vi "mod_Continuous BB-PSK generation.vi"(0 "bit stream type":T4(tab), 1 "Symbol Rate, Hz":dbl=1.0 format="%.2f", 2 "Custom-PSK Parameters":T3 {"PSK type" items=["normal", "shifted", "offset"]; "symbol map" format="%.3f"}, 5 "PN Sequence Order":i32=9, 9 "user base bit pattern":i8[](array[numeric]), 11 "error in (no error)":errorcluster, 12 "filter parameters":T1={"Alpha"=0.5, "Filter Length"=6, "TX Filter"=enum."Root Raised Cos"} {"Alpha" format="%.2f"}, 13 "Path":path) -> (4 "output complex waveform":T2 {"Y" format="%.3f"; "dt" format="%^.2e"; "t0" format="%.4f"}, 6 "samples per symbol":i32, 15 "error out":errorcluster)   [LabVIEW 2020, in "niDMT.lvlib"]
uses:
  <vilib>/addons/Modulation/niDMT.lvlib
  <vilib>/addons/Modulation/Digital/Support/Controls/PSK System Parameters.ctl
  <vilib>/addons/Modulation/Analog/controls/Complex Data Waveform.ctl
  <vilib>/addons/Modulation/Digital/General/MT Generate Bits (Galois, PN Order).vi
  <vilib>/addons/Modulation/Digital/Support/Common/Validators/mod_Generate Bits Validate.vi
  <vilib>/addons/Modulation/Analog/support/mod_Set Error Source.vi
  <vilib>/addons/Modulation/Digital/General/subVIs/mod_Generate Bits PN Sequence.vi
  <vilib>/addons/Modulation/Digital/General/MT Generate Bits (User Defined).vi
  <vilib>/Utility/file.llb/Read From Spreadsheet File (DBL).vi
  <vilib>/addons/Modulation/Digital/Support/Common/Validators/mod_Generate Filter Coefficients Validate.vi
  <vilib>/addons/Modulation/Digital/General/subVIs/mod_Generate Filter Coefficients.vi
  <vilib>/addons/Modulation/niAMT.lvlib
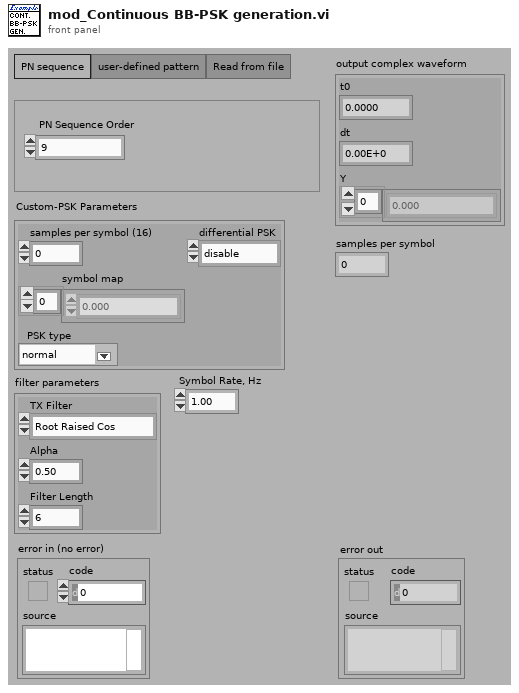
[diagram p1: front panel]
types:
  T1 = cluster{"Alpha":dbl, "Filter Length":i32, "TX Filter":enum16{"none", "Raised Cosine", "Root Raised Cos", "Gaussian"}}
  T2 = typedef "niAMT.lvlib/Complex Data Waveform.ctl" = cluster{"t0":dbl, "dt":dbl, "Y":cdb[]}
  T3 = typedef "niDMT.lvlib/PSK System Parameters.ctl" = cluster{"samples per symbol (16)":i32, "symbol map":cdb[], "differential PSK":enum16{"disable", "enable"}, "PSK type":u16}
  T4 = enum32{"PN sequence", "user-defined pattern", "Read from file"}
  T5 = enum16{"none", "Raised Cosine", "Root Raised Cos", "Gaussian"}
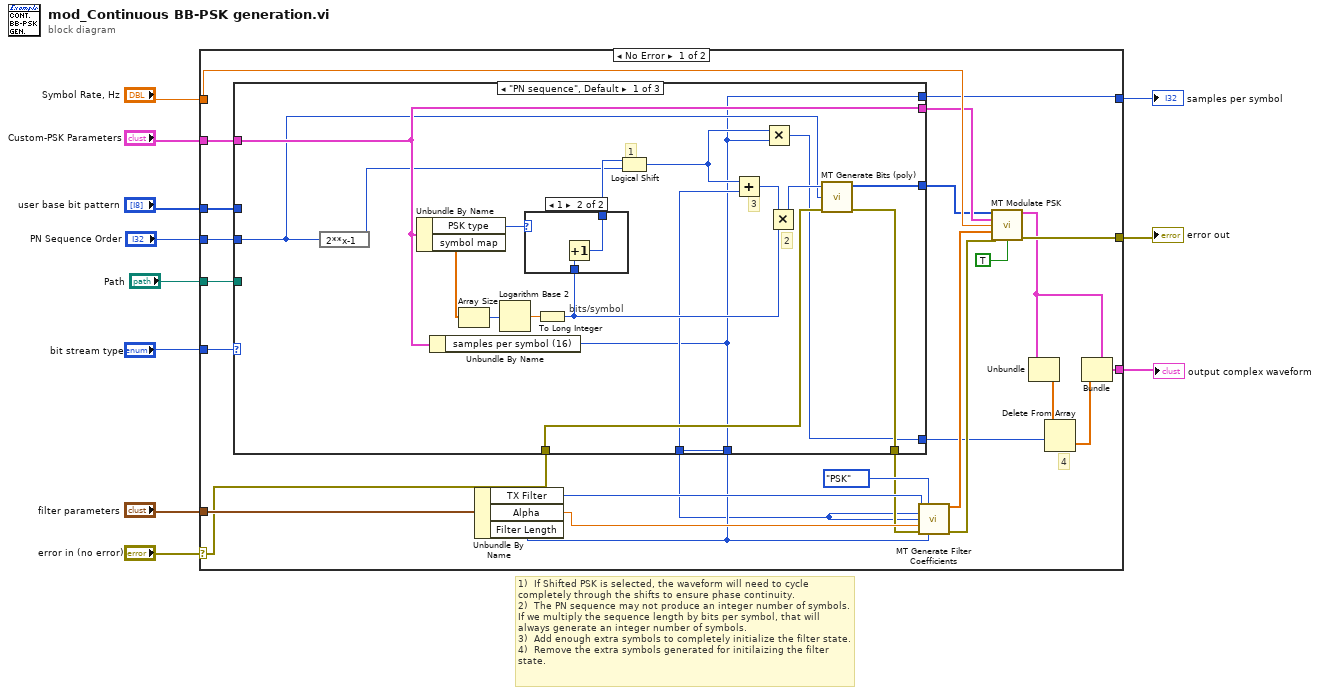
[diagram p0: block diagram]
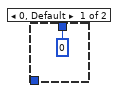
[diagram p2: hidden frame]
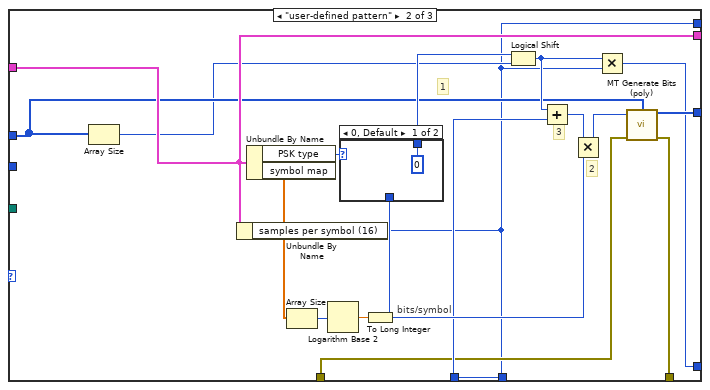
[diagram p3: hidden frame]
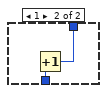
[diagram p4: hidden frame]
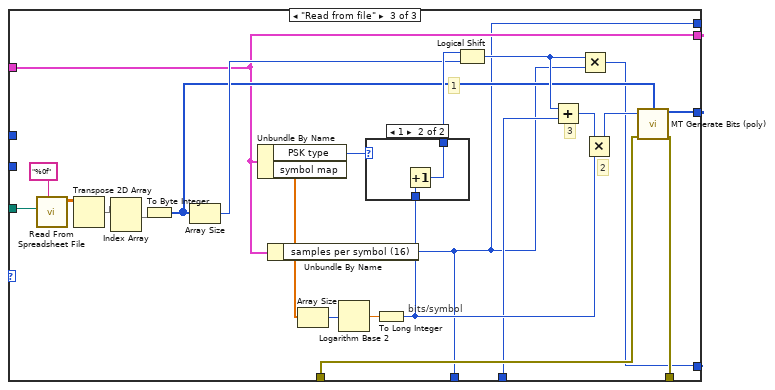
[diagram p5: hidden frame]
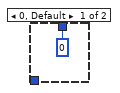
[diagram p6: hidden frame]
diagram:
  # "1)  If Shifted PSK is selected, the waveform will need to cycle completely through the shifts to ensure phase continuity. \n2)  The PN sequence may not produce an integer number of symbols.  If we multiply the sequence length by bits per symbol, that will always generate an integer number of symbols. \n3)  Add enough extra symbols to completely initialize the filter state.\n4)  Remove the extra symbols generated for initilaizing the filter state."
  n1 = case shown="No Error" "error in (no error)" {
    selector: "error in (no error)" -> [w14 w106]
    tunnel: [w13 _] -> w11
    tunnel: [w37 _] -> w10
    tunnel: [w36 w106] -> w9
    tunnel: "Symbol Rate, Hz" -> [w33 _]
    tunnel: "PN Sequence Order" -> [w23 _]
    tunnel: "Custom-PSK Parameters" -> [w21 _]
    tunnel: "user base bit pattern" -> [w32 _]
    tunnel: "bit stream type" -> [w25 _]
    tunnel: "filter parameters" -> [w31 _]
    tunnel: "Path" -> [w24 _]
    frame No Error {
      # "4"
      n2 = Unbundle By Name(w31) -> ("TX Filter"=w34:T5, "Alpha"=w35:dbl, "Filter Length"=w19:i32)
      n3 = case shown="\"PN sequence\", Default" w25 {
        tunnel: w32 -> [_ w65 _]
        tunnel: w24 -> [_ _ w98]
        tunnel: w23 -> [w39 _ _]
        tunnel: w21 -> [w46 w67 w82]
        tunnel: [w46 w67 w82] -> w20
        tunnel: w19 -> [w41 w66 w83]
        tunnel: [w44 w64 w85] -> w18
        tunnel: [w40 w63 w80] -> w17
        tunnel: [w42 w62 w84] -> w15
        tunnel: w14 -> [w45 w61 w86]
        tunnel: [w38 w59 w81] -> w13
        tunnel: [w38 w59 w81] -> w12
        frame "PN sequence", Default {
          # "2"
          # "1"
          # "3"
          # "bits/symbol"
          n4 = expression code="2**x-1"(w39) -> (w43:i32)
          n5 = Unbundle By Name(w46) -> ("PSK type"=w47:u16, "symbol map"=w48:cdb[])
          n6 = Unbundle By Name(w46) -> ("samples per symbol (16)"=w38:i32)
          n7 = Array Size(array=w48) -> (size(s)=w50:i32)
          n8 = Logarithm Base 2(1:w50) -> (0:w51:dbl)
          n9 = To Long Integer(number=w51) -> (32bit integer=w53:i32)
          n10 = case shown="1" w47 {
            tunnel: w53 -> [_ w58]
            tunnel: [0 w57] -> w52
            frame 0, Default {
            }
            frame 1 {
              n11 = Increment(x=w58) -> (x+1=w57:i32)
            }
          }
          n12 = Logical Shift(y=w52, x=w43) -> (x << y=w49:i32)
          n13 = Add(x=w49, y=w41) -> (x+y=w54:i32)
          n14 = Multiply(x=w49, y=w38) -> (x*y=w42:i32)
          n15 = Multiply(x=w54, y=w53) -> (x*y=w55:i32)
          n16 = call-poly <vilib>:"MT Generate Bits (poly).vi"("total bits (128)"=w55, "PN sequence order (9)"=w39, "error in (no error)"=w45) -> ("output bit stream"=w40:i8[], "error out"=w44:errorcluster)  [unwired: 2 in, 9 out]
        }
        frame "user-defined pattern" {
          # "2"
          # "1"
          # "3"
          # "bits/symbol"
          n17 = Array Size(array=w65) -> (size(s)=w60:i32)
          n18 = Unbundle By Name(w67) -> ("samples per symbol (16)"=w59:i32)
          n19 = Unbundle By Name(w67) -> ("PSK type"=w68:u16, "symbol map"=w69:cdb[])
          n20 = Array Size(array=w69) -> (size(s)=w71:i32)
          n21 = Logarithm Base 2(1:w71) -> (0:w72:dbl)
          n22 = To Long Integer(number=w72) -> (32bit integer=w74:i32)
          n23 = case shown="0, Default" w68 {
            tunnel: w74 -> [_ w79]
            tunnel: [0 w78] -> w73
            frame 0, Default {
            }
            frame 1 {
              n24 = Increment(x=w79) -> (x+1=w78:i32)
            }
          }
          n25 = Logical Shift(y=w73, x=w60) -> (x << y=w70:i32)
          n26 = Add(x=w70, y=w66) -> (x+y=w75:i32)
          n27 = Multiply(x=w75, y=w74) -> (x*y=w76:i32)
          n28 = Multiply(x=w70, y=w59) -> (x*y=w62:i32)
          n29 = call-poly <vilib>:"MT Generate Bits (poly).vi"("total bits (128)"=w76, "user base bit pattern"=w65, "error in (no error)"=w61) -> ("output bit stream"=w63:i8[], "error out"=w64:errorcluster)  [unwired: 1 in, 10 out]
        }
        frame "Read from file" {
          # "2"
          # "1"
          # "3"
          # "bits/symbol"
          n30 = call-poly <vilib>:"Read From Spreadsheet File.vi"("format (%.3f)"="%0f", "file path (dialog if empty)"=w98) -> ("all rows"=w100:dbl[][])  [unwired: 2 in, 7 out]
          n31 = Transpose 2D Array(2D array=w100) -> (transposed array=w101:dbl[][])
          n32 = Index Array(array=w101) -> (element=w102:dbl[])  [unwired: 2 in]
          n33 = To Byte Integer(number=w102) -> (8bit integer=w87:i8[])
          n34 = Array Size(array=w87) -> (size(s)=w88:i32)
          n35 = Unbundle By Name(w82) -> ("PSK type"=w89:u16, "symbol map"=w90:cdb[])
          n36 = Unbundle By Name(w82) -> ("samples per symbol (16)"=w81:i32)
          n37 = Array Size(array=w90) -> (size(s)=w92:i32)
          n38 = Logarithm Base 2(1:w92) -> (0:w93:dbl)
          n39 = To Long Integer(number=w93) -> (32bit integer=w95:i32)
          n40 = case shown="1" w89 {
            tunnel: w95 -> [_ w105]
            tunnel: [0 w104] -> w94
            frame 0, Default {
            }
            frame 1 {
              n41 = Increment(x=w105) -> (x+1=w104:i32)
            }
          }
          n42 = Logical Shift(y=w94, x=w88) -> (x << y=w91:i32)
          n43 = Add(x=w91, y=w83) -> (x+y=w96:i32)
          n44 = Multiply(x=w91, y=w81) -> (x*y=w84:i32)
          n45 = Multiply(x=w96, y=w95) -> (x*y=w97:i32)
          n46 = call-poly <vilib>:"MT Generate Bits (poly).vi"("total bits (128)"=w97, "user base bit pattern"=w87, "error in (no error)"=w86) -> ("output bit stream"=w80:i8[], "error out"=w85:errorcluster)  [unwired: 1 in, 10 out]
        }
      }
      n47 = call <vilib>:"MT Generate Filter Coefficients.vi"("pulse shaping filter (none)"=w34, "modulation type"=enum16{"FSK", "PSK", "QAM", "MSK", "PAM", "ASK"}."PSK", "pulse shaping samples per symbol (16)"=w12, "matched samples per symbol (16)"=w12, "filter parameter"=w35, "error in (no error)"=w18, "filter length (symbols)"=w19) -> ("pulse shaping filter coefficients"=w28:dbl[], "error out"=w16:errorcluster)  [unwired: 7 out]
      n48 = call <vilib>:"MT Modulate PSK.vi"("input bit stream"=w17, "PSK system parameters"=w20, "symbol rate (Hz)"=w33, "pulse shaping filter coefficients"=w28, "error in (no error)"=w16, "reset? (T)"=TRUE ("Reset (T)")) -> ("output complex waveform"=w30:T2, "error out"=w36:errorcluster)  [unwired: 1 in, 7 out]
      n49 = Unbundle(w30) -> ("Y"=w26:cdb[])  [unwired: 2 out]
      n50 = Delete From Array(array=w26, length=w15) -> (deleted portion=w27:cdb[])  [unwired: 1 in, 1 out]
      n51 = Bundle(cluster=w30, "Y"=w27) -> (w37:T2)  [unwired: 2 out]
    }
    frame Error {
    }
  }
  "error out" <- w9
  "output complex waveform" <- w10
  "samples per symbol" <- w11
